vi "ClimberSensorStatus.vi"(3 "OperatorControlBox Connected":bool, 4 "OperatorControlBox Buttons":T1, 5 "Raise Complete":bool, 6 "Sensors":T2) -> (0 "MidWheelHit":bool, 1 "FrontWheelHit":bool, 2 "RaiseComplete":bool)   [LabVIEW 2018]
uses:
  TypeDefs/RobotComponents/RobotSensors.ctl
  ArgosLib/Config/ConfigComponents/TypeDefs/Config_DigitalIO.ctl
  <vilib>/Rock Robotics/SystemInterfaces/DIO/FPGA_DIOChannel.ctl
  General/OperatorControlBox/TypeDefs/OperatorControlBoxButtons_Type.ctl
  ArgosLib/Signal Processing/TypeDefs/EdgeDetector_Type.ctl
  ArgosLib/ArgosLib.lvlib
panel:
  in  "ManualRaiseComplete":bool
  in  "ManualMidWheelHit":bool
  in  "ManualFrontWheelHit":bool
  in  "Manual Override":bool
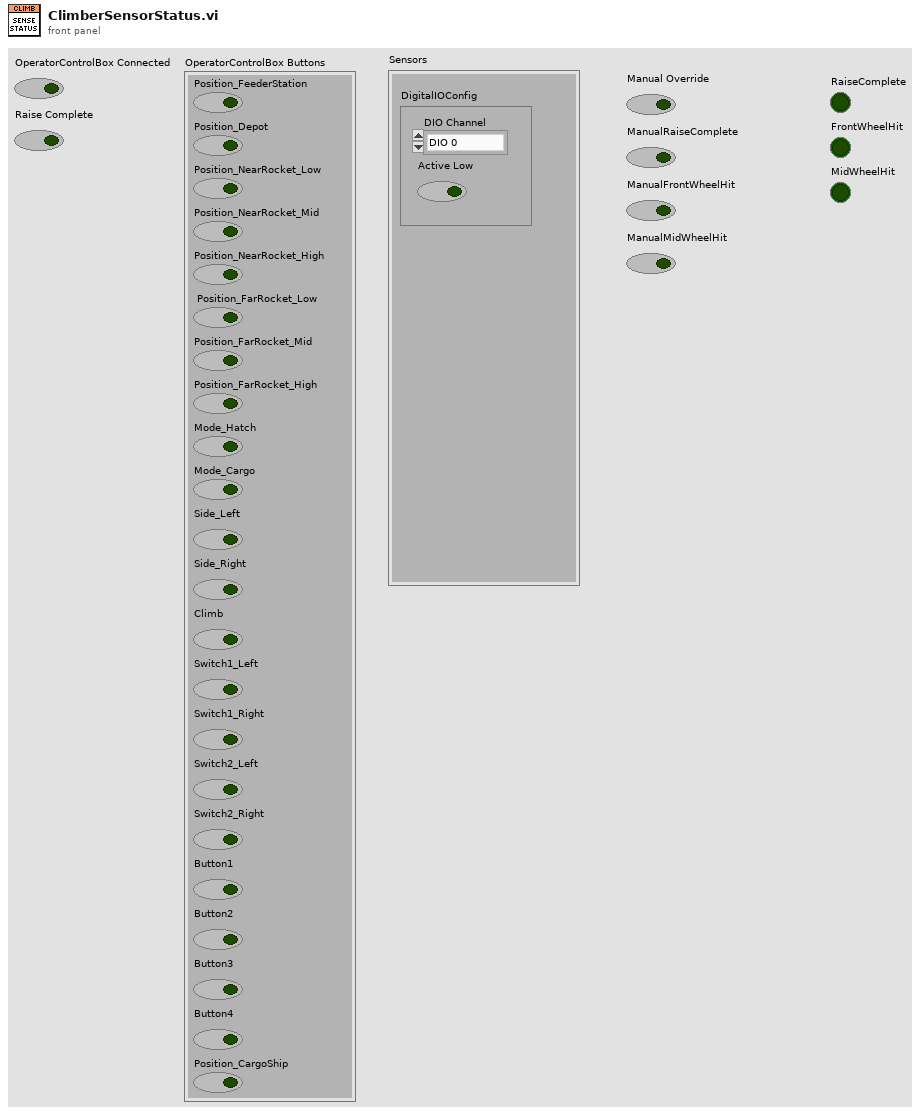
[diagram p1: front panel]
types:
  T1 = typedef "OperatorControlBoxButtons_Type.ctl" = cluster{"Position_FeederStation":bool, "Position_Depot":bool, "Position_NearRocket_Low":bool, "Position_NearRocket_Mid":bool, "Position_NearRocket_High":bool, " Position_FarRocket_Low":bool, "Position_FarRocket_Mid":bool, "Position_FarRocket_High":bool, "Mode_Hatch":bool, "Mode_Cargo":bool, "Side_Left":bool, "Side_Right":bool, "Climb":bool, "Switch1_Left":bool, "Switch1_Right":bool, "Switch2_Left":bool, "Switch2_Right":bool, "Button1":bool, "Button2":bool, "Button3":bool, "Button4":bool, "Position_CargoShip":bool}
  T2 = typedef "RobotSensors.ctl" = cluster{"DigitalIOConfig":T3}
  T3 = typedef "ArgosLib.lvlib/Config_DigitalIO.ctl" = cluster{"DIOChannel":T4, "Active Low":bool}
  T4 = typedef "FPGA_DIOChannel.ctl" = enum8{"DIO 0", "DIO 1", "DIO 2", "DIO 3", "DIO 4", "DIO 5", "DIO 6", "DIO 7", "DIO 8", "DIO 9", "DIO MXP 0", "DIO MXP 1", "DIO MXP 2", "DIO MXP 3", "DIO MXP 4", "DIO MXP 5", "DIO MXP 6", "DIO MXP 7", "DIO MXP 8", "DIO MXP 9", "DIO MXP 10", "DIO MXP 11", "DIO MXP 12", "DIO MXP 13", "DIO MXP 14", "DIO MXP 15", "SPI Port CS1", "SPI Port CS2", "SPI Port CS3", "SPI Port MISO", "SPI Port MOSI", "Invalid"}
  T5 = typedef "ArgosLib.lvlib/EdgeDetector_Type.ctl" = enum16{"RisingEdge", "FallingEdge", "Both"}
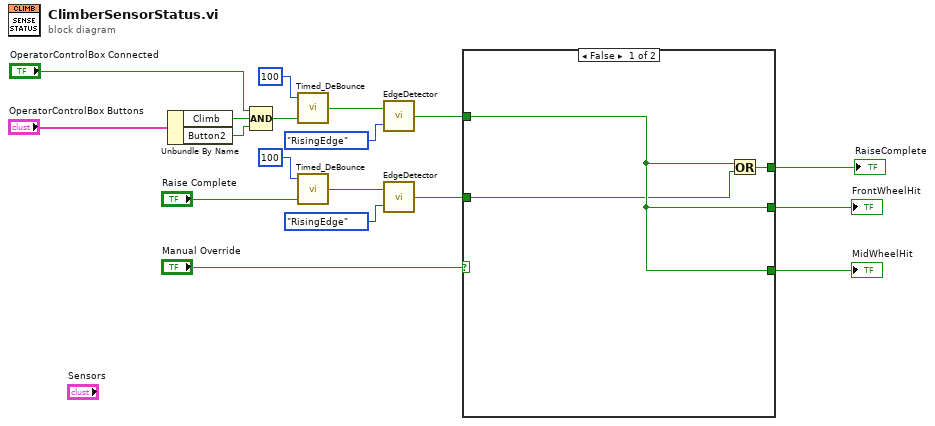
[diagram p0: block diagram]
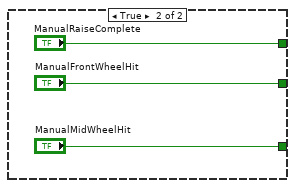
[diagram p2: hidden frame]
diagram:
  n1 = Unbundle By Name("OperatorControlBox Buttons") -> ("Climb"=w12:bool, "Button2"=w11:bool)
  n2 = Compound Arithmetic op=AND("OperatorControlBox Connected", w12, w11) -> (w10:bool)
  n3 = call "Timed_DeBounce.vi"("Input"=w10, "Hold Time(ms)"=u32 100) -> ("Output"=w9:bool)  [unwired: 1 in]
  n4 = call "Timed_DeBounce.vi"("Input"="Raise Complete", "Hold Time(ms)"=u32 100) -> ("Output"=w3:bool)  [unwired: 1 in]
  n5 = call "EdgeDetector.vi"("DetectorType"=EdgeDetector_Type."RisingEdge", "Input"=w9) -> ("Edge"=w6:bool)
  n6 = call "EdgeDetector.vi"("DetectorType"=EdgeDetector_Type."RisingEdge", "Input"=w3) -> ("Edge"=w1:bool)
  n7 = case shown="False" "Manual Override" {
    tunnel: [w21 "ManualFrontWheelHit"] -> w18
    tunnel: [w21 "ManualMidWheelHit"] -> w17
    tunnel: [w20 "ManualRaiseComplete"] -> w15
    tunnel: w6 -> [w21 _]
    tunnel: w1 -> [w19 _]
    frame False {
      n8 = Or(x=w21, y=w19) -> (x .or. y?=w20:bool)
    }
    frame True {
    }
  }
  "FrontWheelHit" <- w18
  "MidWheelHit" <- w17
  "RaiseComplete" <- w15
